vi "tb_interpolation_fft_simio_compile.vi"() -> ()   [LabVIEW 2011]
uses:
  <vilib>/Platform/TimedLoop/XDataNode/XDataNode.xnode
  <vilib>/Platform/TimedLoop/XDataNode/nitl_modes.ctl
  <vilib>/Platform/TimedLoop/XDataNode/XDNodeRunTimeDep.lvlib
  <vilib>/Platform/TimedLoop/XDataNode/wakeup.ctl
  <vilib>/Platform/TimedLoop/XDataNode/timing_clust.ctl
  <vilib>/rvi/DataTransferAndStorage/Container/XNode/niFpgaContainer.xnode
  <vilib>/rvi/FXPMathLib/FxpInterpret/XNode/nifxpmath_Interpret.xnode
  <vilib>/eio/EIONode/EIONode.xnode
  <userlib>/FPGA Library/Code Development/Signal Processing/Interpolation Block/Controls/Interpolation Input Data.ctl
  <vilib>/rvi/FXPMathLib/basic elements/FxpDiscreteDelay/XNode/nifxpmath_DiscreteDelay.xnode
  <vilib>/rvi/FIFO/Fifo_Resource/nirvififoEmulationRead.vi
  <vilib>/rvi/FIFO/Fifo_Resource/nirvififoEmulationWrite.vi
  <vilib>/rvi/FIFO/Fifo_Resource/nirvififoEmulationGetNumberOfElementsToRead.vi
  <vilib>/rvi/eio/common/nirviEmuTemplateMethod_errors.vi
  <vilib>/rvi/interface/RandomDataEmulation/nirviRandomDataFpgaReadWriteTemplate.vi
  <userlib>/FPGA Library/Code Development/Signal Processing/FFT Block/FFT/Controls/FFT States.ctl
  <userlib>/FPGA Library/Code Development/Signal Processing/FFT Block/FFT/Controls/FFT Parameters.ctl
panel:
  out "Interp Loop Overflow":bool
  out "Current FFT State":T1
  out "FFT Status":T2
  in  "Address":u32
  in  "Data":T3 {"x[n].ResampleInfo"."Lambda" format="%.18g"; "x[n-1].ResampleInfo"."Lambda" format="%.18g"}
  in  "Write?":bool
  in  "FFT Parameters":T4={"Direction"=TRUE, "scale_sch"=85.0, "Flush Length"=0} {"scale_sch" format="%.0b"}
  in  "FFT State":cluster{"FFT State":T1, "Set FFT State?":bool}
  out "acq timed out?":bool
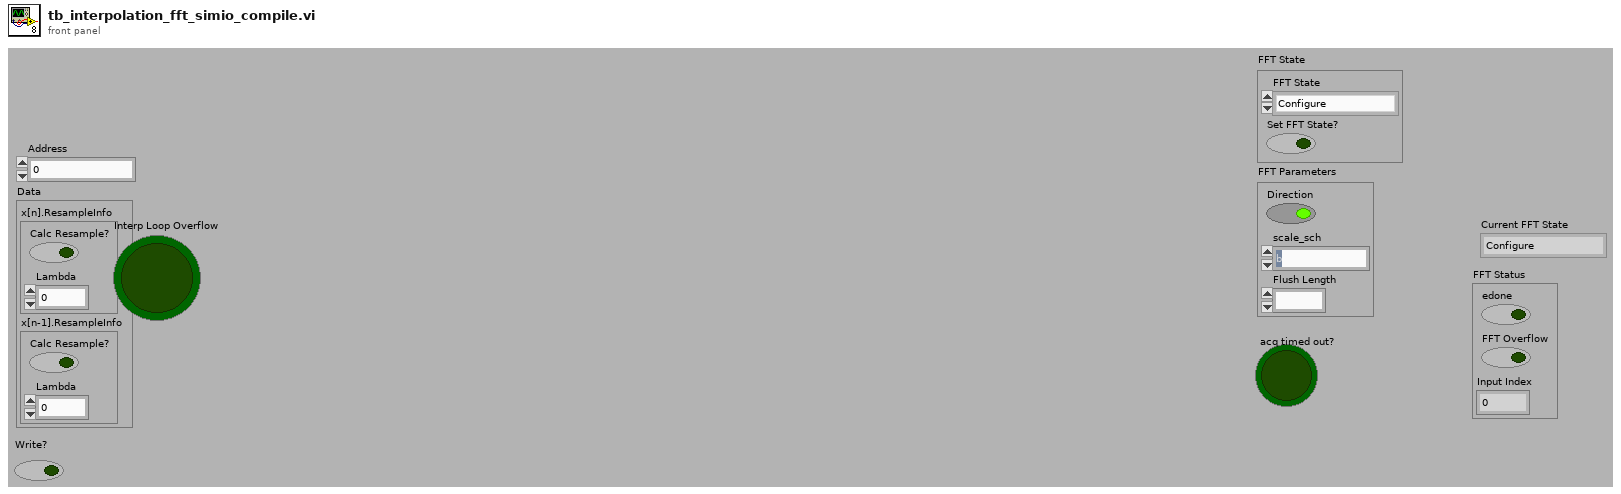
[diagram p1: front panel]
types:
  T1 = typedef "FFT States.ctl" = enum8{"Configure", "Start FFT processing", "Process", "Unload Last FFT", "Reset"}
  T2 = cluster{"edone":bool, "FFT Overflow":bool, "Input Index":fxp<+,9,9>}
  T3 = cluster{"x[n].ResampleInfo":cluster{"Calc Resample?":bool, "Lambda":fxp<+/-,18,1>}, "x[n-1].ResampleInfo":cluster{"Calc Resample?":bool, "Lambda":fxp<+/-,18,1>}}
  T4 = typedef "FFT Parameters.ctl" = cluster{"Direction":bool, "scale_sch":fxp<+,10,10>, "Flush Length":u16}
  T5 = typedef "XDNodeRunTimeDep.lvlib/timing_clust.ctl" = cluster{"Expected End [f-1]":u64, "Actual End [f-1]":u64, "Finished Late? [f-1]":bool, "Expected End [i-1]":u64, "Actual End [i-1]":u64, "Finished Late? [i-1]":bool, "Expected Start [i]":u64, "Actual Start [i]":u64, "Expected Start [f]":u64, "Actual Start [f]":u64, "Source Name":string, "Structure Name":string, "Period":i64, "Deadline":i64, "Offset":i64, "Start":i64, "Priority":i32, "Timeout":i32, "Mode":T6, "Wakeup Reason":T7, "Error":errorcluster, "Source Type":string, "Secondary Source Type":string, "Global End Time":u64, "Global Start Time":u64, "Frame Duration":u64, "Iteration Duration":u64, "Assigned CPU":i32, "I/O Scan Engine Mode":u32}
  T6 = typedef "XDNodeRunTimeDep.lvlib/nitl_modes.ctl" = enum32{"No Change", "Process missed periods, maintain original phase", "Discard missed periods, maintain original phase", "Process missed periods, ignore original phase", "Discard missed periods, ignore original phase"}
  T7 = typedef "XDNodeRunTimeDep.lvlib/wakeup.ctl" = enum32{"Normal", "Aborted", "Asynchronous wakeup", "Timing source error", "Timed loop error", "Timeout"}
  T8 = typedef "Interpolation Input Data.ctl" = fxp<+/-,18,1>
  T9 = typedef "Interpolation Output Data.ctl" = fxp<+/-,19,1>
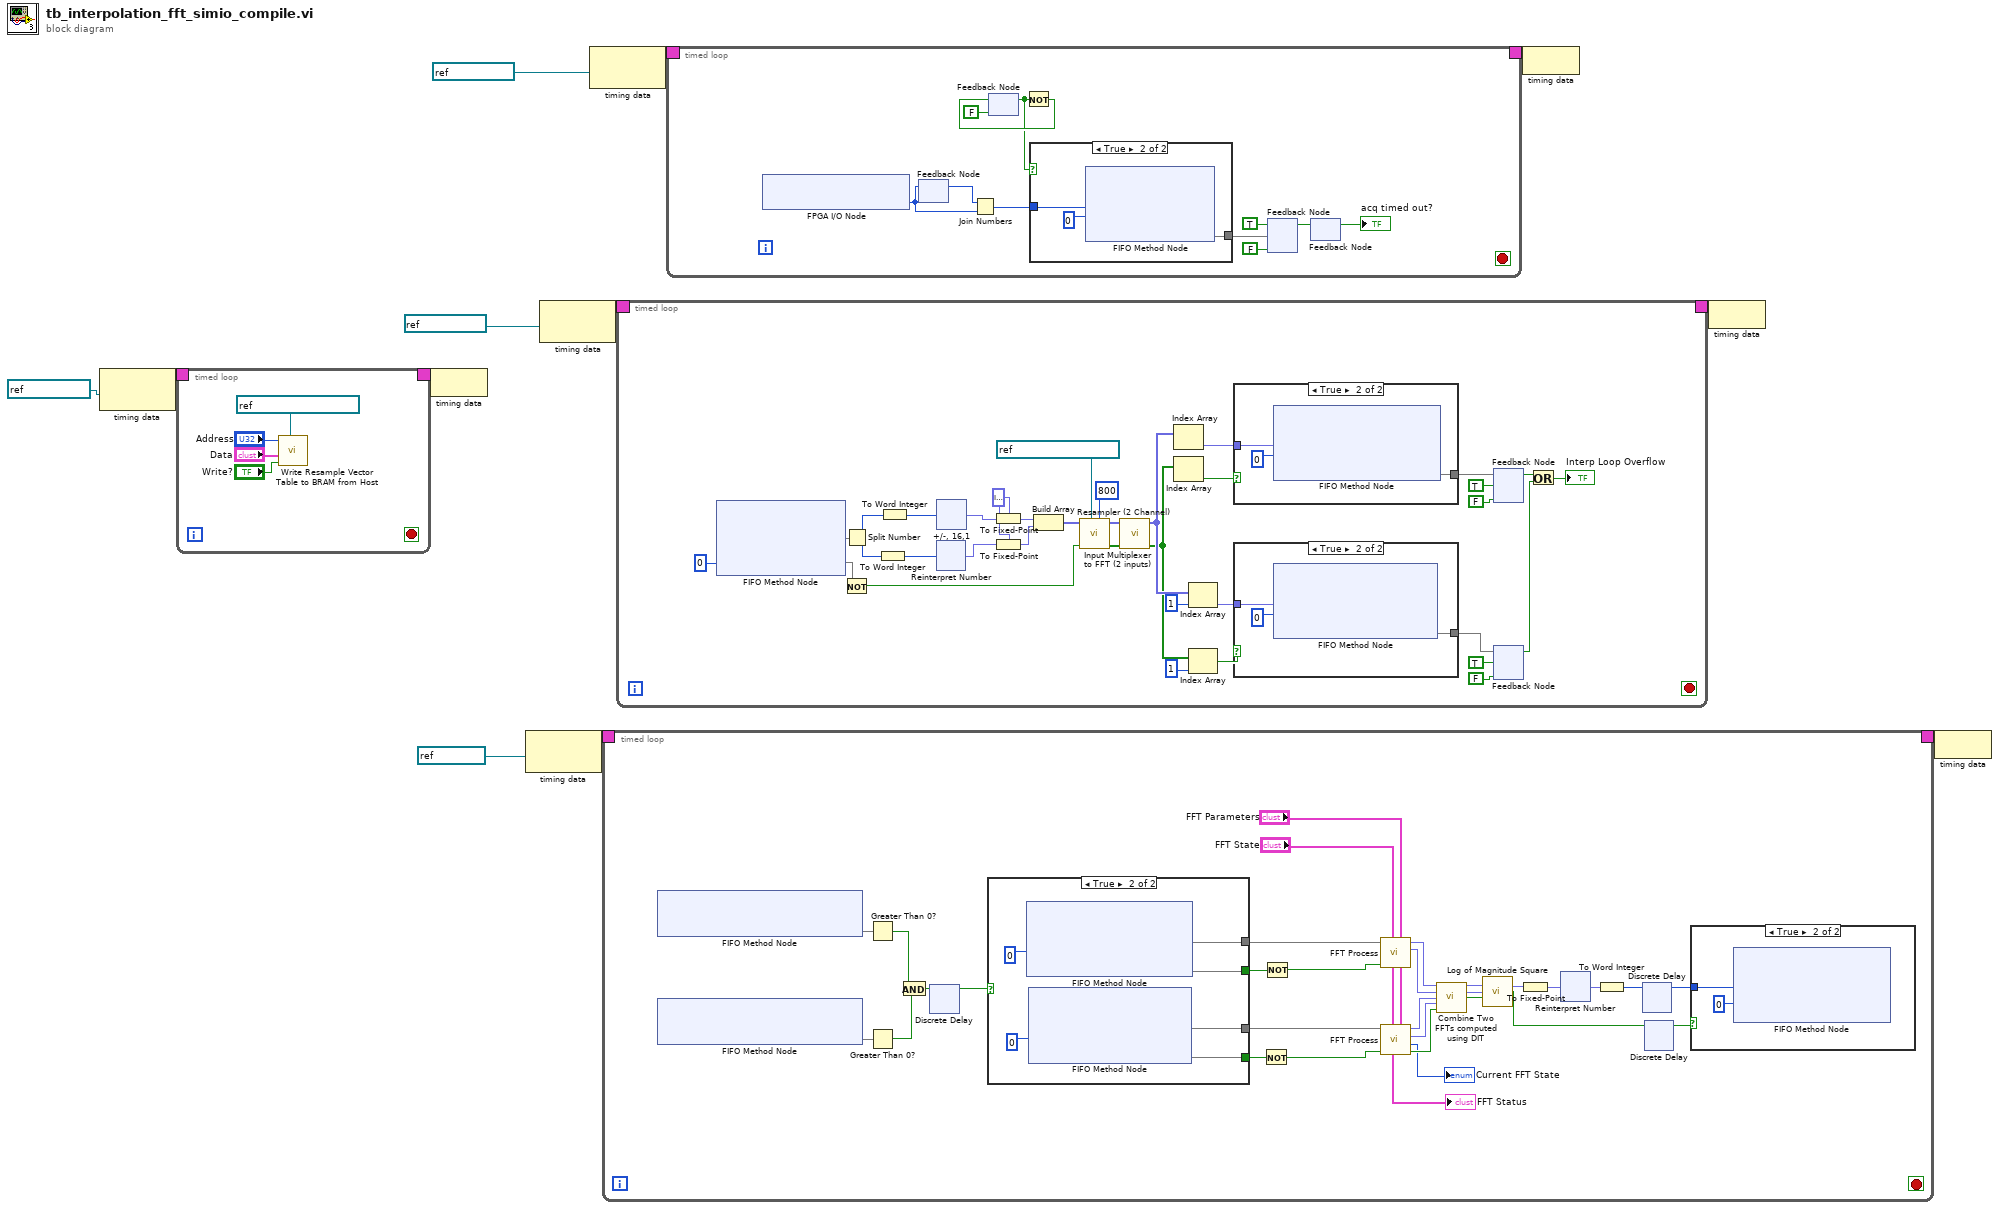
[diagram p0: block diagram]
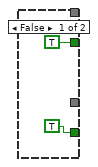
[diagram p6: hidden frame]
diagram:
  n1 = node-c288(refnum<k21> "126.67MHz" ("Source Name")) -> (w6:T5)
  n2 = timed-loop {
    timing: w6 -> [_]
    timing-out: [_] -> w5
    stop <- _ stop-if-true
    n3 = call <userlib>:"Write Resample Vector Table to BRAM from Host.vi"("Resample Table"=refnum<k21> "Interpolation Table", "Write?"="Write?", "Data"="Data", "Address"="Address") -> ()  [unwired: 8 in]
  }
  n4 = node-c288(w5) -> ()
  n5 = node-c288(refnum<k21> "250MHz" ("Source Name")) -> (w12:T5)
  n6 = node-c288(refnum<k21> "126.67MHz" ("Source Name")) -> (w3:T5)
  n7 = node-c288(refnum<k21> "ADC Clock" ("Source Name")) -> (w10:T5)
  n8 = timed-loop {
    timing: w12 -> [_]
    timing-out: [_] -> w11
    stop <- _ stop-if-true
    n9 = xnode ("FIFO Method Node")() -> ("Number of Elements to Read"=w45)  [unwired: 1 in, 1 out]
    n10 = xnode ("FIFO Method Node")() -> ("Number of Elements to Read"=w44)  [unwired: 1 in, 1 out]
    n11 = Greater Than 0?(x=w45) -> (x > 0?=w43:bool)
    n12 = Greater Than 0?(x=w44) -> (x > 0?=w42:bool)
    n13 = And(x=w43, y=w42) -> (x .and. y?=w41:bool)
    n14 = xnode "Discrete Delay"("D"=w41) -> ("Q"=w19:bool)
    n15 = case shown="True" w19 {
      tunnel: [TRUE ("Timed Out?") w57] -> w49
      tunnel: [_ w56] -> w24
      tunnel: [_ w55] -> w23
      tunnel: [TRUE ("Timed Out?") w54] -> w48
      frame False {
      }
      frame True {
        n16 = xnode ("FIFO Method Node")("Timeout"=0) -> ("Element"=w56, "Timed Out?"=w57)  [unwired: 1 in, 1 out]
        n17 = xnode ("FIFO Method Node")("Timeout"=0) -> ("Element"=w55, "Timed Out?"=w54)  [unwired: 1 in, 1 out]
      }
    }
    n18 = Not(x=w48) -> (.not. x?=w25:bool)
    n19 = Not(x=w49) -> (.not. x?=w46:bool)
    n20 = call <userlib>:"FFT Process.vi"("FFT Parameters"="FFT Parameters", "FFT State"="FFT State", "Input Valid"=w46, "Real Data In"=w24) -> ("Imag Data Out"=w37:fxp<+/-,16,1>, "Real Data Out"=w38:fxp<+/-,16,1>)  [unwired: 2 in, 4 out]
    n21 = call <userlib>:"FFT Process.vi"("FFT Parameters"="FFT Parameters", "FFT State"="FFT State", "Input Valid"=w25, "Real Data In"=w23) -> ("Output Valid"=w31:bool, "Current FFT State"=→"Current FFT State":T1, "Imag Data Out"=w35:fxp<+/-,16,1>, "Real Data Out"=w36:fxp<+/-,16,1>, "FFT Status"=→"FFT Status":T2)  [unwired: 2 in, 1 out]
    n22 = call <userlib>:"Combine Two FFTs computed using DIT.vi"("Real FFT 1"=w38, "Imag FFT 1"=w37, "Real FFT 2"=w36, "Imag FFT 2"=w35, "Input Data Valid"=w31) -> ("Real FFT k"=w28:fxp<+/-,24,3>, "Imag FFT k"=w27:fxp<+/-,24,3>, "Output Valid"=w26:bool)  [unwired: 6 in, 2 out]
    n23 = call <userlib>:"Log of Magnitude Square.vi"("Real"=w28, "Imaginary"=w27, "Input Valid"=w26) -> ("Log Magnitude"=w21:fxp<+/-,34,12>, "Output Valid"=w39:bool)  [unwired: 11 in]
    n24 = To Fixed-Point(number=w21) -> (fixed-point=w29:fxp<+/-,16,8>)  [unwired: 1 in]
    n25 = xnode "Reinterpret Number"("x"=w29) -> ("y"=w47:fxp<+/-,16,16>)
    n26 = To Word Integer(number=w47) -> (16bit integer=w40:i16)
    n27 = xnode "Discrete Delay"("D"=w40) -> ("Q"=w20:i16)
    n28 = xnode "Discrete Delay"("D"=w39) -> ("Q"=w22:bool)
    n29 = case shown="True" w22 {
      tunnel: w20 -> [_ w51]
      frame False {
      }
      frame True {
        n30 = xnode ("FIFO Method Node")("Element"=w51, "Timeout"=0) -> ()  [unwired: 1 in, 2 out]
      }
    }
  }
  n31 = timed-loop {
    timing: w3 -> [_]
    timing-out: [_] -> w2
    stop <- _ stop-if-true
    w79 = T8 0.0 ("Interpolate.Input Data")
    n32 = xnode ("FIFO Method Node")("Timeout"=0) -> ("Element"=w82, "Timed Out?"=w77)  [unwired: 1 in, 1 out]
    n33 = Not(x=w77) -> (.not. x?=w71:bool)
    n34 = Split Number(x=w82) -> (hi(x)=w70:u16, lo(x)=w69:u16)
    n35 = To Word Integer(number=w69) -> (16bit integer=w67:i16)
    n36 = To Word Integer(number=w70) -> (16bit integer=w68:i16)
    n37 = xnode "Reinterpret Number"("x"=w67) -> ("y"=w75:fxp<+/-,16,1>)
    n38 = xnode "+/-, 16,1"("x"=w68) -> ("y"=w73:fxp<+/-,16,1>)
    n39 = To Fixed-Point(fixed-point type=w79, number=w73) -> (fixed-point=w74:T8)
    n40 = To Fixed-Point(fixed-point type=w79, number=w75) -> (fixed-point=w80:T8)
    n41 = Build Array(w74, w80) -> (w78:T8[])
    n42 = call <userlib>:"Resampler (2 Channel).vi"("CalibrationTable Length-1"=u16 800, "ResampleVectorInfo"=refnum<k21> "Interpolation Table", "DataValid"=w71, "Input Data"=w78) -> ("Data Valid"=w100:bool[], "Interpolated Data"=w101:T9[])  [unwired: 6 in]
    n43 = call <userlib>:"Input Multiplexer to FFT (2 inputs).vi"("Input Data Valid Array"=w100, "Input Data"=w101) -> ("Output Data Valid Array"=w95:bool[], "Interchanged Data"=w97:T9[])  [unwired: 8 in]
    n44 = Index Array(array=w97) -> (element=w99:T9)  [unwired: 1 in]
    n45 = Index Array(array=w95) -> (element=w98:bool)  [unwired: 1 in]
    n46 = Index Array(array=w97, index=1) -> (element=w96:T9)
    n47 = Index Array(array=w95, index=1) -> (element=w94:bool)
    n48 = case shown="True" w98 {
      tunnel: w99 -> [_ w111]
      tunnel: [_ w109] -> w91
      frame False {
      }
      frame True {
        n49 = xnode ("FIFO Method Node")("Element"=w111, "Timeout"=0) -> ("Timed Out?"=w109)  [unwired: 1 in, 1 out]
      }
    }
    n50 = case shown="True" w94 {
      tunnel: w96 -> [_ w108]
      tunnel: [_ w106] -> w88
      frame False {
      }
      frame True {
        n51 = xnode ("FIFO Method Node")("Element"=w108, "Timeout"=0) -> ("Timed Out?"=w106)  [unwired: 1 in, 1 out]
      }
    }
    n52 = feedback-in #1(w91, TRUE) -> ()
    n53 = feedback #1(FALSE ("Timed Out?")) -> (w87:bool)
    n54 = feedback #2(FALSE ("Timed Out?")) -> (w84:bool)
    n55 = feedback-in #2(w88, TRUE) -> ()
    n56 = Or(x=w87, y=w84) -> (x .or. y?=→"Interp Loop Overflow":bool)
  }
  n57 = timed-loop {
    timing: w10 -> [_]
    timing-out: [_] -> w9
    stop <- _ stop-if-true
    n58 = xnode "FPGA I/O Node"() -> ("IO Module\\AI 0 Data"=w115:i16)  [unwired: 1 in, 1 out]
    n59 = feedback-in #3(w115) -> ()
    n60 = feedback #3() -> (w116:i16)  [unwired: 1 in]
    n61 = Join Numbers(hi=w116, lo=w115) -> ((hi.lo)=w117:u32)
    n62 = feedback #4(FALSE) -> (w118:bool)
    n63 = Not(x=w118) -> (.not. x?=w124:bool)
    n64 = feedback-in #4(w124) -> ()
    n65 = case shown="True" w118 {
      tunnel: w117 -> [_ w127]
      tunnel: [_ w125] -> w121
      frame False {
      }
      frame True {
        n66 = xnode ("FIFO Method Node")("Element"=w127, "Timeout"=0) -> ("Timed Out?"=w125)  [unwired: 1 in, 1 out]
      }
    }
    n67 = feedback-in #5(TRUE, w121) -> ()
    n68 = feedback #5(FALSE) -> (w119:bool)
    n69 = feedback-in #6(w119) -> ()
    n70 = feedback #6() -> (→"acq timed out?":bool)  [unwired: 1 in]
  }
  n71 = node-c288(w9) -> ()
  n72 = node-c288(w2) -> ()
  n73 = node-c288(w11) -> ()
